vi "中水三立数据传输UI.vi"() -> ()   [LabVIEW 2016, in "中水三立SQL数据传输.lvlib"]
panel:
  in  "开机启动":bool
  out "数据大小":i32
  out "数据上传中":bool
  out "当前时间":timestamp
  out "error out":errorcluster
  out "数据查表起始时间":cluster{"dbo.LS_Data":string}
  in  "数据补传":bool caption="确定"
  out "读取报文显示":string
  out "发送报文显示":string
  out "通信状态":bool
  in  "配置信息":T1
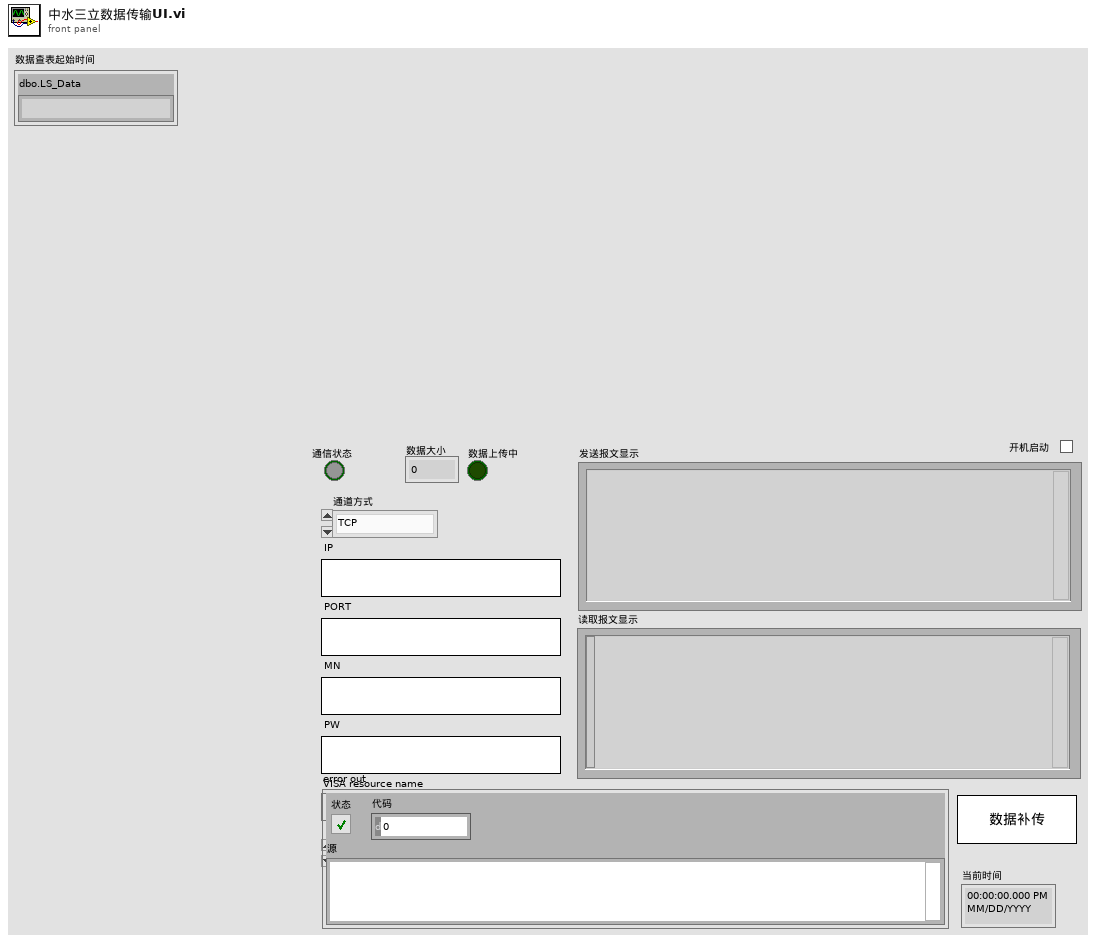
[diagram p1: front panel]
types:
  T1 = cluster{"通道方式":enum16{"TCP", "serial"}, "IP":string, "PORT":string, "MN":string, "PW":string, "VISA resource name":refnum<visa-resource-name>, "baud rate":u32}
  T2 = typedef "LVDateTimeRec.ctl" = cluster{"秒数的小数部分":dbl, "秒":i32, "分":i32, "时":i32, "日":i32, "月":i32, "年":i32, "天数（周）":i32, "天数（年）":i32, "DST":i32}
  T3 = cluster{"枚举":enum16{"打开连接", "发送数据", "读取数据", "数据处理", "关闭连接"}, "data":string}
  T4 = cluster{"枚举":enum16{"TCP", "serial"}, "IP":string, "PORT":string, "MN":string, "PW":string, "VISA resource name":refnum<visa-resource-name>, "baud rate":u32}
  T5 = typedef "中水三立SQL数据传输.lvlib/data_in.ctl" = cluster{"PW":string, "MN":string, "table输入":T6, "数据发送次数":i32, "枚举":enum16{"返回请求应答", "上传数据", "返回执行结果"}, "type":T7, "因子编码&数据类型":cluster{"因子编码":string, "数据类型":string}[]}
  T6 = typedef "中水三立SQL数据传输.lvlib/table.ctl" = string
  T7 = typedef "中水三立SQL数据传输.lvlib/Type.ctl" = string
  T8 = cluster{"table":string, "columns":string[], "condition":string, "data_in":T5}
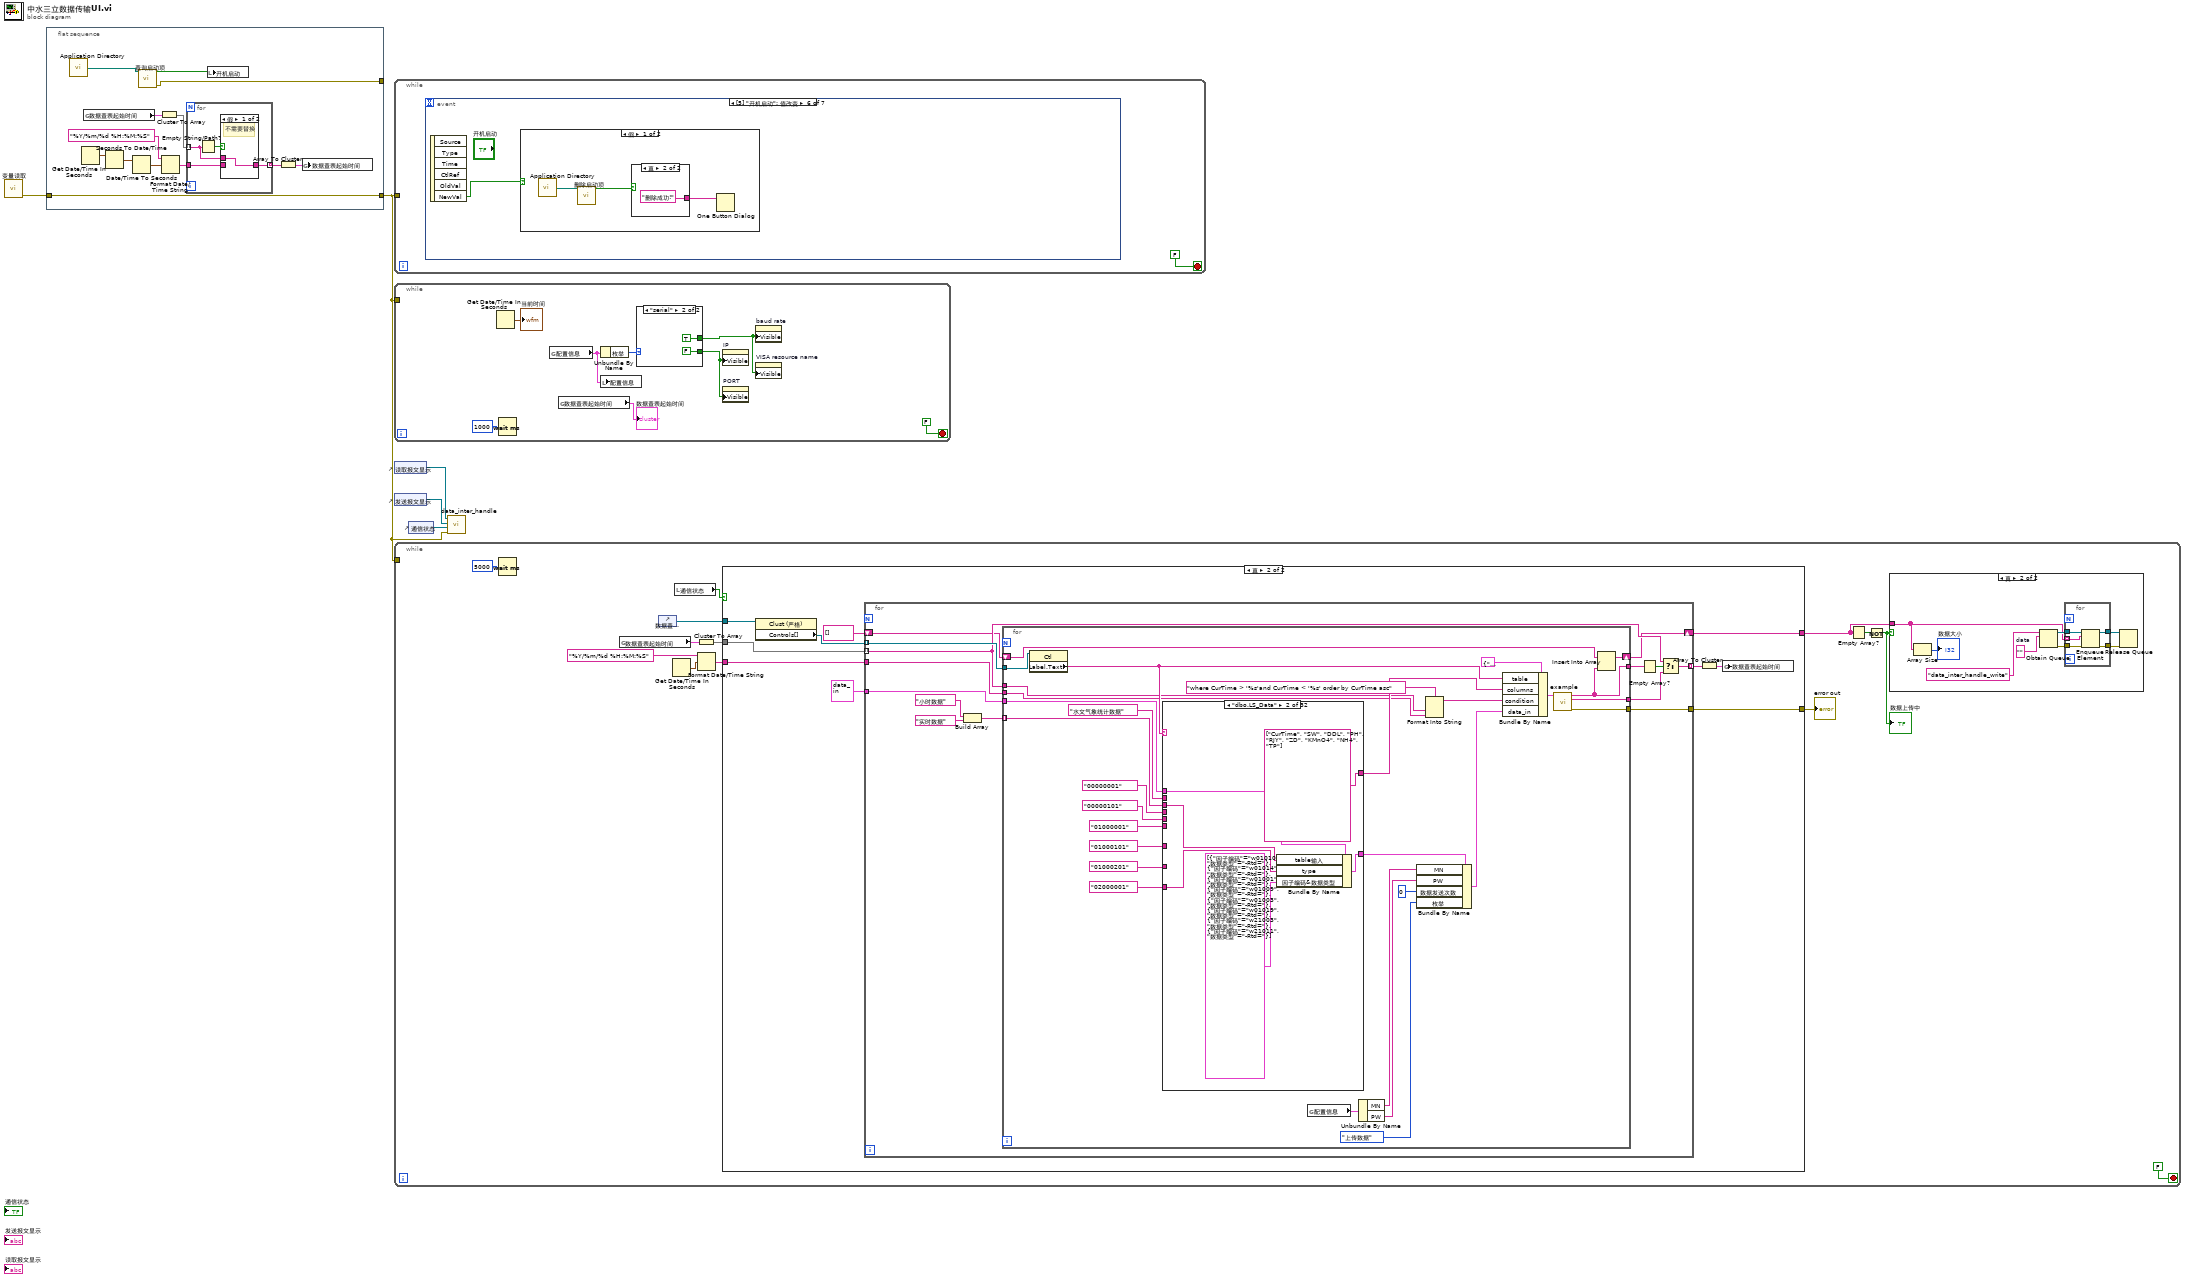
[diagram p0: block diagram]
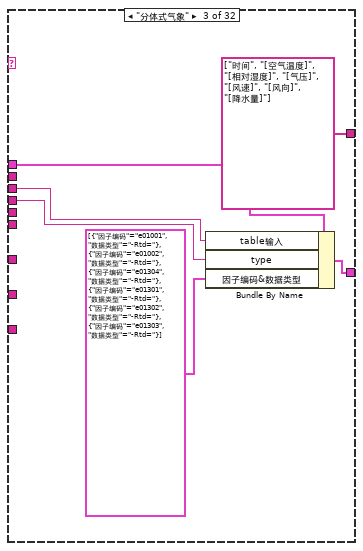
[diagram p5: hidden frame]
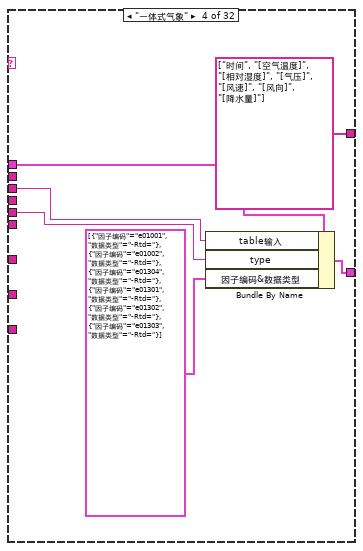
[diagram p6: hidden frame]
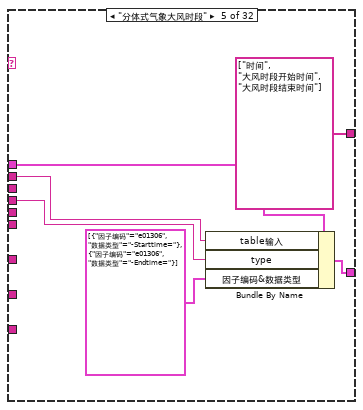
[diagram p7: hidden frame]
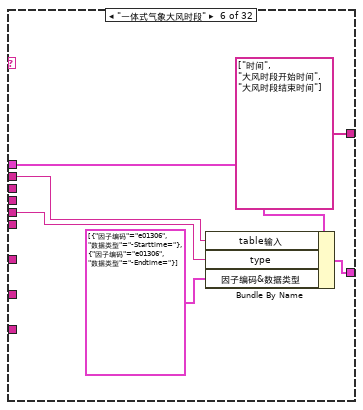
[diagram p8: hidden frame]
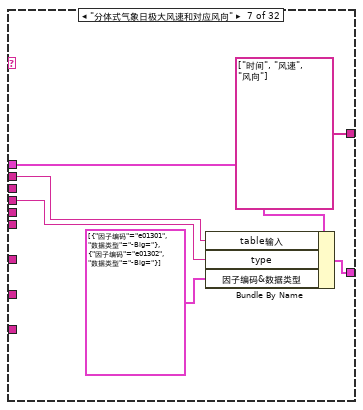
[diagram p9: hidden frame]
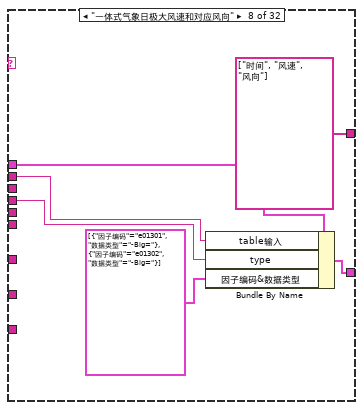
[diagram p10: hidden frame]
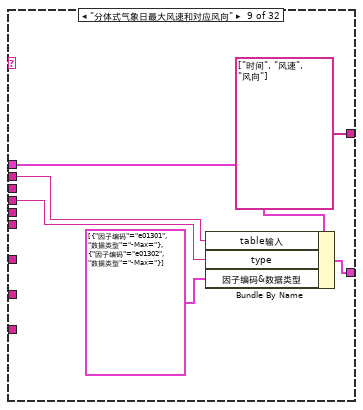
[diagram p11: hidden frame]
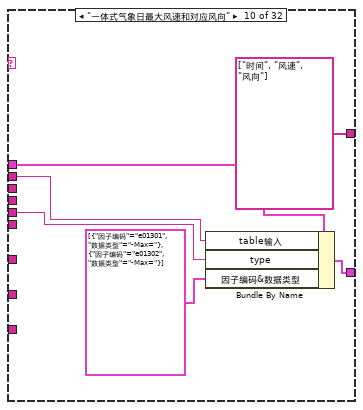
[diagram p12: hidden frame]
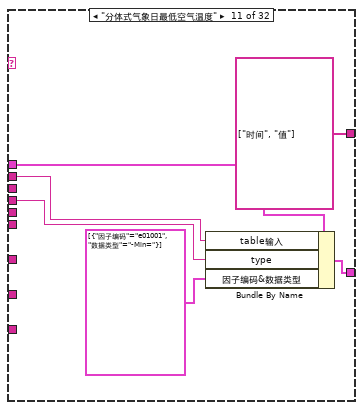
[diagram p13: hidden frame]
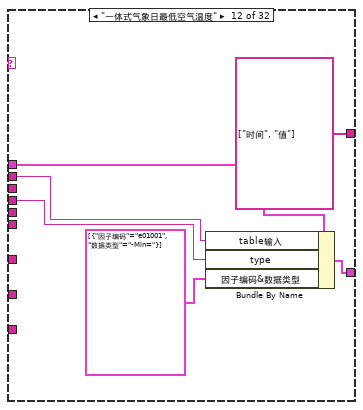
[diagram p14: hidden frame]
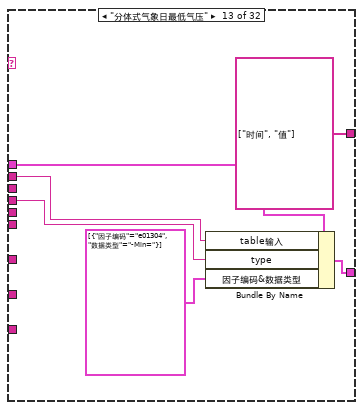
[diagram p15: hidden frame]
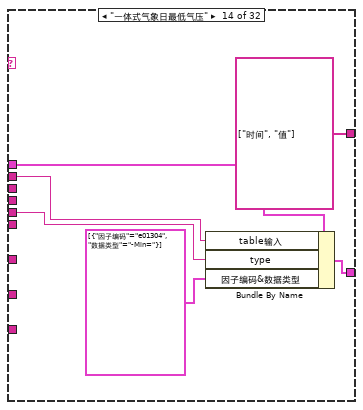
[diagram p16: hidden frame]
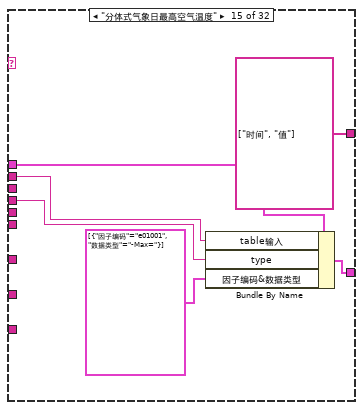
[diagram p17: hidden frame]
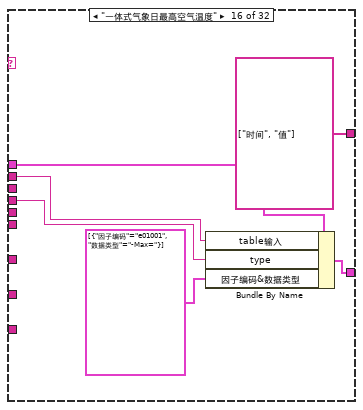
[diagram p18: hidden frame]
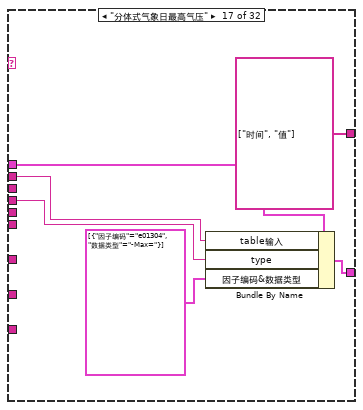
[diagram p19: hidden frame]
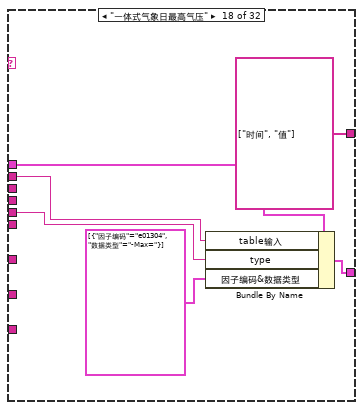
[diagram p20: hidden frame]
diagram:
  n1 = call "变量读取.vi"() -> ("错误输出"=w5:errorcluster)  [unwired: 11 in]
  n2 = flat-sequence {
    tunnel: w5 -> [w11]
    tunnel: [w11] -> w4
    tunnel: [w6] -> _
    frame #0 {
      n3 = call <vilib>:"Application Directory.vi"() -> ("Application Directory"=w8:path)
      n4 = Get Date/Time In Seconds() -> (seconds since 1Jan1904=w10:timestamp)
      n5 = global read "断电保存全局.vi" "数据查表起始时间"() -> (w16:cluster{"dbo.LS_Data":string})
      n6 = Seconds To Date/Time(time stamp (now)=w10) -> (date time rec=w9:T2)  [unwired: 1 in]
      n7 = Date/Time To Seconds(2:w9) -> (0:w14:timestamp)  [unwired: 1 in]
      n8 = call "查询启动项.vi"("启动文件路径"=w8) -> ("error out"=w6:errorcluster, "包含启动项"=w7:bool)  [unwired: 9 in]
      n9 = Cluster To Array(cluster=w16) -> (array=w17:string[])
      n10 = Format Date/Time String(time format string (%c)="%Y/%m/%d %H:%M:%S" ("时间格式字符串(%c)"), seconds (now)=w14) -> (date/time string=w13:string)  [unwired: 1 in]
      n11 = for {
        tunnel: w17 -> [w19] mode=indexing
        tunnel: w13 -> [w21]
        tunnel: [w20] -> w18 mode=indexing
        n12 = Empty String/Path?(string/path=w19) -> (empty?=w22:bool)
        n13 = case shown="假" w22 {
          tunnel: w21 -> [_ w24]
          tunnel: [w23 w24] -> w20
          tunnel: w19 -> [w23 _]
          frame False {
            # "不需要替换"
          }
          frame True {
            # "空字符串，替换"
          }
        }
      }
      n14 = local write "开机启动"(w7) -> ()
      n15 = Array To Cluster(array=w18) -> (cluster=w12:cluster{"[0]":string})
      n16 = global write "断电保存全局.vi" "数据查表起始时间"(w12) -> ()
    }
  }
  n17 = while {
    tunnel: w4 -> [_]
    stop <- FALSE stop-if-true
    n18 = event shown="[5] \"开机启动\": 值改变" {
      selector: _ -> [_ _ _ _ _ _ _]
      dyn-events: _ -> [_ _ _ _ _ _ _]
      timeout: _ -> [_ _ _ _ _ _ _]
      event Timeout {
        n19 = event-data() -> ()  [unwired: 1 in, 3 out]
      }
      event "配置信息.IP", "配置信息.PORT": Mouse Down {
        n20 = event-data() -> ("CtlRef"=w34:refnum<vi>)  [unwired: 1 in, 7 out]
        n21 = property class="Str"(reference=w34) -> (reference out=w27:refnum<vi>, "Value"=w33:string)  [unwired: 1 in, 1 out]
        n22 = call "IP键盘.vi"("OldNumber"=w33) -> ("NewNumber"=w26:string)
        n23 = String Length(string=w26) -> (length=w32:i32)
        n24 = Less Or Equal?(x=w32, y=50) -> (x <= y?=w30:bool)
        n25 = case shown="假" w30 {
          tunnel: w27 -> [w35 w39]
          tunnel: w26 -> [_ w38]
          tunnel: [w35 w39] -> w29
          tunnel: ["127.0.0.1" w38] -> w28
          frame False {
            n26 = One Button Dialog(message="超过ipv4最大长度限制,请重新输入!" ("消息")) -> ()  [unwired: 1 in, 1 out]
          }
          frame True {
          }
        }
        n27 = property class="Str"(reference=w29, "Val(Sgnl)"=w28) -> ()  [unwired: 1 in, 2 out]
      }
      event "配置信息.baud rate": Mouse Down {
        n28 = event-data() -> ("CtlRef"=w43:refnum<vi>)  [unwired: 1 in, 7 out]
        n29 = property class="DigNum (严格)"(reference=w43) -> (reference out=w41:refnum<vi>, "Value"=w42:u32)  [unwired: 1 in, 1 out]
        n30 = call "数字键盘.vi"("OldNumber"=w42) -> ("NewNumber"=w40:sgl)
        n31 = property class="DigNum (严格)"(reference=w41, "Val(Sgnl)"=w40) -> ()  [unwired: 1 in, 2 out]
      }
      event "配置信息": Value Change {
        n32 = event-data() -> ()  [unwired: 1 in, 6 out]
        n33 = flat-sequence {
          frame #0 {
            n34 = global write "断电保存全局.vi" "配置信息"("配置信息") -> ()
          }
          frame #1 {
            w49 = T3 {"枚举"=enum."打开连接", "data"=""}
            n35 = call "变量存储.vi"() -> ()  [unwired: 12 in]
            n36 = Bundle By Name(cluster=w49, "枚举"=enum16{"打开连接", "发送数据", "读取数据", "数据处理", "关闭连接"}."关闭连接") -> (w48:T3)
            n37 = Obtain Queue(name (unnamed)="data_inter_handle" ("名称（未命名）"), element data type=w49) -> (queue out=w51:refnum<queue>, error out=w50:errorcluster)  [unwired: 3 in, 1 out]
            n38 = Enqueue Element(queue=w51, element=w48, error in (no error)=w50) -> (queue out=w45:refnum<queue>, error out=w46:errorcluster)  [unwired: 1 in, 1 out]
            n39 = Release Queue(queue=w45, error in (no error)=w46) -> ()  [unwired: 1 in, 3 out]
          }
        }
      }
      event "数据补传": Value Change {
        n40 = event-data() -> ()  [unwired: 1 in, 6 out]
        n41 = call "数据补传对话框.vi"() -> ("输出"=w54:bool, "时间OUT"=w53:timestamp)  [unwired: 10 in]
        n42 = case shown="真" w54 {
          tunnel: w53 -> [_ w59]
          frame False {
          }
          frame True {
            n43 = Format Date/Time String(time format string (%c)="%Y/%m/%d %H:%M:%S" ("时间格式字符串(%c)"), seconds (now)=w59) -> (date/time string=w56:string)  [unwired: 1 in]
            n44 = Initialize Array(w56, 1 ("维数大小")) -> (w55:string[])
            n45 = Array To Cluster(array=w55) -> (cluster=w57:cluster{"[0]":string})
            n46 = global write "断电保存全局.vi" "数据查表起始时间"(w57) -> ()
          }
        }
      }
      event "开机启动": Value Change {
        n47 = event-data() -> ("NewVal"=w61:bool)  [unwired: 1 in, 5 out]
        n48 = case shown="假" w61 {
          frame False {
            n49 = call <vilib>:"Application Directory.vi"() -> ("Application Directory"=w63:path)
            n50 = call "删除启动项.vi"("启动文件路径"=w63) -> ("删除标记"=w62:bool)  [unwired: 9 in, 1 out]
            n51 = case shown="真" w62 {
              tunnel: ["删除失败!" "删除成功!"] -> w64
              frame False {
              }
              frame True {
              }
            }
            n52 = One Button Dialog(message=w64) -> ()  [unwired: 1 in, 1 out]
          }
          frame True {
            n53 = call <vilib>:"Application Directory.vi"() -> ("Application Directory"=w69:path)
            n54 = call "添加启动项.vi"("启动文件路径"=w69) -> ("添加成功标记"=w68:bool)  [unwired: 9 in, 1 out]
            n55 = case shown="假" w68 {
              tunnel: ["添加失败!" "添加成功!"] -> w67
              frame False {
              }
              frame True {
              }
            }
            n56 = One Button Dialog(message=w67) -> ()  [unwired: 1 in, 1 out]
          }
        }
      }
      event Panel Close {
        n57 = event-data() -> ()  [unwired: 1 in, 4 out]
        n58 = Quit LabVIEW(quit? (T)=TRUE ("退出？(T)")) -> ()
      }
    }
  }
  n59 = while {
    tunnel: w4 -> [_]
    stop <- FALSE stop-if-true
    n60 = Get Date/Time In Seconds() -> (seconds since 1Jan1904=→"当前时间":timestamp)
    n61 = Wait (ms)(milliseconds to wait=u32 1000 ("等待时间（毫秒）")) -> ()  [unwired: 1 out]
    n62 = global read "断电保存全局.vi" "配置信息"() -> (w76:T4)
    n63 = global read "断电保存全局.vi" "数据查表起始时间"() -> (→"数据查表起始时间":cluster{"dbo.LS_Data":string})
    n64 = local write "配置信息"(w76) -> ()
    n65 = Unbundle By Name(w76) -> ("枚举"=w75:enum16{"TCP", "serial"})
    n66 = case shown="\"serial\"" w75 {
      tunnel: [TRUE FALSE] -> w74
      tunnel: [FALSE TRUE] -> w73
      frame "TCP", Default {
      }
      frame "serial" {
      }
    }
    n67 = property on="IP" class="Str"("Visible"=w74) -> ()  [unwired: 2 in, 2 out]
    n68 = property on="PORT" class="Str"("Visible"=w74) -> ()  [unwired: 2 in, 2 out]
    n69 = property on="baud rate" class="DigNum (严格)"("Visible"=w73) -> ()  [unwired: 2 in, 2 out]
    n70 = property on="VISA resource name" class="VISAName"("Visible"=w73) -> ()  [unwired: 2 in, 2 out]
  }
  n71 = control-ref of="读取报文显示"() -> (w2:refnum<vi>)
  n72 = control-ref of="发送报文显示"() -> (w3:refnum<vi>)
  n73 = while {
    tunnel: w4 -> [_]
    stop <- FALSE stop-if-true
    n74 = Wait (ms)(milliseconds to wait=u32 5000 ("等待时间（毫秒）")) -> ()  [unwired: 1 out]
    n75 = global read "断电保存全局.vi" "数据查表起始时间"() -> (w95:cluster{"dbo.LS_Data":string})
    n76 = control-ref of="数据查表起始时间"() -> (w89:refnum<vi>)
    n77 = Get Date/Time In Seconds() -> (seconds since 1Jan1904=w91:timestamp)
    n78 = local read "通信状态"() -> (w86:bool)
    n79 = Cluster To Array(cluster=w95) -> (array=w94:string[])
    n80 = Format Date/Time String(time format string (%c)="%Y/%m/%d %H:%M:%S" ("时间格式字符串(%c)"), seconds (now)=w91) -> (date/time string=w92:string)  [unwired: 1 in]
    n81 = case shown="真" w86 {
      tunnel: w94 -> [_ w107]
      tunnel: w92 -> [_ w106]
      tunnel: [_ w105] -> w85
      tunnel: w89 -> [_ w104]
      tunnel: [_ w102] -> w88
      frame False {
      }
      frame True {
        n82 = property class="Clust (严格)"(reference=w104) -> ("Controls[]"=w103:refnum<vi>[])  [unwired: 1 in, 2 out]
        n83 = for {
          tunnel: w107 -> [w117] mode=indexing
          tunnel: w103 -> [w121] mode=indexing
          tunnel: w106 -> [w120]
          shift-right: [w108] -> w105
          shift-left: string[] [] ("message") -> [w109]
          tunnel: [w115] -> w99 mode=indexing
          tunnel: [w114] -> w102
          tunnel: T5 {"PW"="123456", "MN"="TEST001", "table输入"="心跳包", "数据发送次数"=0, "枚举"=enum."上传数据", "type"="00000001", "因子编码&数据类型"=[{"因子编码"="e01306", "数据类型"="-Starttime="}, {"因子编码"="e01307", "数据类型"="-Endtime="}]} ("data_in") -> [w113]
          n84 = Build Array(T6 "小时数据" ("table输入"), T6 "实时数据" ("table输入")) -> (w110:T6[])
          n85 = for {
            tunnel: w121 -> [w151]
            tunnel: w120 -> [w140]
            tunnel: [w123] -> w119
            tunnel: w117 -> [w138]
            tunnel: [w137] -> w116
            tunnel: [w136] -> w114
            tunnel: w113 -> [w134]
            tunnel: w110 -> [w125] mode=indexing
            shift-right: [w122] -> w108
            shift-left: w109 -> [w124]
            n86 = property class="Ctl"(reference=w151) -> ("Label.Text"=w150:string)  [unwired: 1 in, 2 out]
            n87 = case shown="\"dbo.LS_Data\"" w150 {
              tunnel: [_ string[] ["CurTime", "SW", "DDL", "PH", "RJY", "ZD", "KMnO4", "NH4", "TP"] ("columns") string[] ["时间", "[空气温度]", "[相对湿度]", "[气压]", "[风速]", "[风向]", "[降水量]"] ("columns") string[] ["时间", "[空气温度]", "[相对湿度]", "[气压]", "[风速]", "[风向]", "[降水量]"] ("columns") string[] ["时间", "大风时段开始时间", "大风时段结束时间"] ("columns") string[] ["时间", "大风时段开始时间", "大风时段结束时间"] ("columns") string[] ["时间", "风速", "风向"] ("columns") string[] ["时间", "风速", "风向"] ("columns") string[] ["时间", "风速", "风向"] ("columns") string[] ["时间", "风速", "风向"] ("columns") string[] ["时间", "值"] ("columns") string[] ["时间", "值"] ("columns") string[] ["时间", "值"] ("columns") string[] ["时间", "值"] ("columns") string[] ["时间", "值"] ("columns") string[] ["时间", "值"] ("columns") string[] ["时间", "值"] ("columns") string[] ["时间", "值"] ("columns") string[] ["时间", "值"] ("columns") string[] ["时间", "值"] ("columns") string[] ["时间", "值"] ("columns") string[] ["时间", "值"] ("columns") string[] ["时间", "[60秒能见度]"] ("columns") string[] ["时间", "[潮高]"] ("columns") string[] ["时间", "[潮高]"] ("columns") string[] ["时间", "[潮高]"] ("columns") string[] ["时间", "[潮高]"] ("columns") string[] ["时间", "[潮高]"] ("columns") string[] ["时间", "[潮高]"] ("columns") string[] ["时间", "[潮高]"] ("columns") string[] ["时间", "[潮高]"] ("columns") string[] ["时间", "[潮高]"] ("columns")] -> w149
              tunnel: w134 -> [_ w156 w162 w168 w174 w180 w186 w192 w198 w204 w210 w216 w222 w228 w234 w240 w246 w252 w258 w264 w270 w276 w282 w288 w294 w300 w306 w312 w318 w324 w330 w336]
              tunnel: [_ w155 w161 w167 w173 w179 w185 w191 w197 w203 w209 w215 w221 w227 w233 w239 w245 w251 w257 w263 w269 w275 w281 w287 w293 w299 w305 w311 w317 w323 w329 w335] -> w148
              tunnel: T7 "00000001" ("type") -> [_ _ w158 _ w171 _ w183 w188 w195 _ w207 w213 w219 _ w231 w237 w243 _ w255 _ w266 _ w278 _ _ _ _ _ _ _ _ _]
              tunnel: T7 "00000101" ("type") -> [_ _ _ w164 _ w176 _ _ _ w201 _ _ _ w225 _ _ _ w249 _ w261 _ w273 _ _ _ _ _ _ _ _ _ _]
              tunnel: T7 "01000001" ("type") -> [_ _ _ _ _ _ _ _ _ _ _ _ _ _ _ _ _ _ _ _ _ _ _ w285 _ _ w302 _ _ w321 _ _]
              tunnel: T7 "01000101" ("type") -> [_ _ _ _ _ _ _ _ _ _ _ _ _ _ _ _ _ _ _ _ _ _ _ _ w291 _ _ w309 _ _ w326 _]
              tunnel: T7 "01000201" ("type") -> [_ _ _ _ _ _ _ _ _ _ _ _ _ _ _ _ _ _ _ _ _ _ _ _ _ w297 _ _ w314 _ _ w333]
              tunnel: T7 "02000001" ("type") -> [_ w152 _ _ _ _ _ _ _ _ _ _ _ _ _ _ _ _ _ _ _ _ _ _ _ _ _ _ _ _ _ _]
              tunnel: w125 -> [_ w153 w159 w165 _ _ _ _ _ _ _ _ _ _ _ _ _ _ _ _ _ _ w279 w284 w290 w296 _ _ _ _ _ _]
              tunnel: T6 "水文气象统计数据" ("table输入") -> [_ _ _ _ w170 w177 w182 w189 w194 w200 w206 w212 w218 w224 w230 w236 w242 w248 w254 w260 w267 w272 _ _ _ _ w303 w308 w315 w320 w327 w332]
              frame "假", Default {
              }
              frame "dbo.LS_Data" {
                n88 = Bundle By Name(cluster=w156, "table输入"=w153, "type"=w152, "因子编码&数据类型"=cluster{"因子编码":string, "数据类型":string}[] [{"因子编码"="w01010", "数据类型"="-Rtd="}, {"因子编码"="w01014", "数据类型"="-Rtd="}, {"因子编码"="w01001", "数据类型"="-Rtd="}, {"因子编码"="w01009", "数据类型"="-Rtd="}, {"因子编码"="w01003", "数据类型"="-Rtd="}, {"因子编码"="w01019", "数据类型"="-Rtd="}, {"因子编码"="w21003", "数据类型"="-Rtd="}, {"因子编码"="w21011", "数据类型"="-Rtd="}]) -> (w155:T5)
              }
              frame "分体式气象" {
                n89 = Bundle By Name(cluster=w162, "table输入"=w159, "type"=w158, "因子编码&数据类型"=cluster{"因子编码":string, "数据类型":string}[] [{"因子编码"="e01001", "数据类型"="-Rtd="}, {"因子编码"="e01002", "数据类型"="-Rtd="}, {"因子编码"="e01304", "数据类型"="-Rtd="}, {"因子编码"="e01301", "数据类型"="-Rtd="}, {"因子编码"="e01302", "数据类型"="-Rtd="}, {"因子编码"="e01303", "数据类型"="-Rtd="}]) -> (w161:T5)
              }
              frame "一体式气象" {
                n90 = Bundle By Name(cluster=w168, "table输入"=w165, "type"=w164, "因子编码&数据类型"=cluster{"因子编码":string, "数据类型":string}[] [{"因子编码"="e01001", "数据类型"="-Rtd="}, {"因子编码"="e01002", "数据类型"="-Rtd="}, {"因子编码"="e01304", "数据类型"="-Rtd="}, {"因子编码"="e01301", "数据类型"="-Rtd="}, {"因子编码"="e01302", "数据类型"="-Rtd="}, {"因子编码"="e01303", "数据类型"="-Rtd="}]) -> (w167:T5)
              }
              frame "分体式气象大风时段" {
                n91 = Bundle By Name(cluster=w174, "table输入"=w170, "type"=w171, "因子编码&数据类型"=cluster{"因子编码":string, "数据类型":string}[] [{"因子编码"="e01306", "数据类型"="-Starttime="}, {"因子编码"="e01306", "数据类型"="-Endtime="}]) -> (w173:T5)
              }
              frame "一体式气象大风时段" {
                n92 = Bundle By Name(cluster=w180, "table输入"=w177, "type"=w176, "因子编码&数据类型"=cluster{"因子编码":string, "数据类型":string}[] [{"因子编码"="e01306", "数据类型"="-Starttime="}, {"因子编码"="e01306", "数据类型"="-Endtime="}]) -> (w179:T5)
              }
              frame "分体式气象日极大风速和对应风向" {
                n93 = Bundle By Name(cluster=w186, "table输入"=w182, "type"=w183, "因子编码&数据类型"=cluster{"因子编码":string, "数据类型":string}[] [{"因子编码"="e01301", "数据类型"="-Big="}, {"因子编码"="e01302", "数据类型"="-Big="}]) -> (w185:T5)
              }
              frame "一体式气象日极大风速和对应风向" {
                n94 = Bundle By Name(cluster=w192, "table输入"=w189, "type"=w188, "因子编码&数据类型"=cluster{"因子编码":string, "数据类型":string}[] [{"因子编码"="e01301", "数据类型"="-Big="}, {"因子编码"="e01302", "数据类型"="-Big="}]) -> (w191:T5)
              }
              frame "分体式气象日最大风速和对应风向" {
                n95 = Bundle By Name(cluster=w198, "table输入"=w194, "type"=w195, "因子编码&数据类型"=cluster{"因子编码":string, "数据类型":string}[] [{"因子编码"="e01301", "数据类型"="-Max="}, {"因子编码"="e01302", "数据类型"="-Max="}]) -> (w197:T5)
              }
              frame "一体式气象日最大风速和对应风向" {
                n96 = Bundle By Name(cluster=w204, "table输入"=w200, "type"=w201, "因子编码&数据类型"=cluster{"因子编码":string, "数据类型":string}[] [{"因子编码"="e01301", "数据类型"="-Max="}, {"因子编码"="e01302", "数据类型"="-Max="}]) -> (w203:T5)
              }
              frame "分体式气象日最低空气温度" {
                n97 = Bundle By Name(cluster=w210, "table输入"=w206, "type"=w207, "因子编码&数据类型"=cluster{"因子编码":string, "数据类型":string}[] [{"因子编码"="e01001", "数据类型"="-Min="}]) -> (w209:T5)
              }
              frame "一体式气象日最低空气温度" {
                n98 = Bundle By Name(cluster=w216, "table输入"=w212, "type"=w213, "因子编码&数据类型"=cluster{"因子编码":string, "数据类型":string}[] [{"因子编码"="e01001", "数据类型"="-Min="}]) -> (w215:T5)
              }
              frame "分体式气象日最低气压" {
                n99 = Bundle By Name(cluster=w222, "table输入"=w218, "type"=w219, "因子编码&数据类型"=cluster{"因子编码":string, "数据类型":string}[] [{"因子编码"="e01304", "数据类型"="-Min="}]) -> (w221:T5)
              }
              frame "一体式气象日最低气压" {
                n100 = Bundle By Name(cluster=w228, "table输入"=w224, "type"=w225, "因子编码&数据类型"=cluster{"因子编码":string, "数据类型":string}[] [{"因子编码"="e01304", "数据类型"="-Min="}]) -> (w227:T5)
              }
              frame "分体式气象日最高空气温度" {
                n101 = Bundle By Name(cluster=w234, "table输入"=w230, "type"=w231, "因子编码&数据类型"=cluster{"因子编码":string, "数据类型":string}[] [{"因子编码"="e01001", "数据类型"="-Max="}]) -> (w233:T5)
              }
              frame "一体式气象日最高空气温度" {
                n102 = Bundle By Name(cluster=w240, "table输入"=w236, "type"=w237, "因子编码&数据类型"=cluster{"因子编码":string, "数据类型":string}[] [{"因子编码"="e01001", "数据类型"="-Max="}]) -> (w239:T5)
              }
              frame "分体式气象日最高气压" {
                n103 = Bundle By Name(cluster=w246, "table输入"=w242, "type"=w243, "因子编码&数据类型"=cluster{"因子编码":string, "数据类型":string}[] [{"因子编码"="e01304", "数据类型"="-Max="}]) -> (w245:T5)
              }
              frame "一体式气象日最高气压" {
                n104 = Bundle By Name(cluster=w252, "table输入"=w248, "type"=w249, "因子编码&数据类型"=cluster{"因子编码":string, "数据类型":string}[] [{"因子编码"="e01304", "数据类型"="-Max="}]) -> (w251:T5)
              }
              frame "分体式气象日最小相对湿度" {
                n105 = Bundle By Name(cluster=w258, "table输入"=w254, "type"=w255, "因子编码&数据类型"=cluster{"因子编码":string, "数据类型":string}[] [{"因子编码"="e01002", "数据类型"="-Min="}]) -> (w257:T5)
              }
              frame "一体式气象日最小相对湿度" {
                n106 = Bundle By Name(cluster=w264, "table输入"=w260, "type"=w261, "因子编码&数据类型"=cluster{"因子编码":string, "数据类型":string}[] [{"因子编码"="e01002", "数据类型"="-Min="}]) -> (w263:T5)
              }
              frame "分体式气象日降水量" {
                n107 = Bundle By Name(cluster=w270, "table输入"=w267, "type"=w266, "因子编码&数据类型"=cluster{"因子编码":string, "数据类型":string}[] [{"因子编码"="e01303", "数据类型"="-Day="}]) -> (w269:T5)
              }
              frame "一体式气象日降水量" {
                n108 = Bundle By Name(cluster=w276, "table输入"=w272, "type"=w273, "因子编码&数据类型"=cluster{"因子编码":string, "数据类型":string}[] [{"因子编码"="e01303", "数据类型"="-Day="}]) -> (w275:T5)
              }
              frame "能见度" {
                n109 = Bundle By Name(cluster=w282, "table输入"=w279, "type"=w278, "因子编码&数据类型"=cluster{"因子编码":string, "数据类型":string}[] [{"因子编码"="e01305", "数据类型"="-Rtd="}]) -> (w281:T5)
              }
              frame "浮子水位计" {
                n110 = Bundle By Name(cluster=w288, "table输入"=w284, "type"=w285, "因子编码&数据类型"=cluster{"因子编码":string, "数据类型":string}[] [{"因子编码"="e01308", "数据类型"="-Rtd="}]) -> (w287:T5)
              }
              frame "雷达水位计" {
                n111 = Bundle By Name(cluster=w294, "table输入"=w290, "type"=w291, "因子编码&数据类型"=cluster{"因子编码":string, "数据类型":string}[] [{"因子编码"="e01308", "数据类型"="-Rtd="}]) -> (w293:T5)
              }
              frame "压力水位计" {
                n112 = Bundle By Name(cluster=w300, "table输入"=w296, "type"=w297, "因子编码&数据类型"=cluster{"因子编码":string, "数据类型":string}[] [{"因子编码"="e01308", "数据类型"="-Rtd="}]) -> (w299:T5)
              }
              frame "浮子水位计低潮" {
                n113 = Bundle By Name(cluster=w306, "table输入"=w303, "type"=w302, "因子编码&数据类型"=cluster{"因子编码":string, "数据类型":string}[] [{"因子编码"="e01310", "数据类型"="-Trough="}]) -> (w305:T5)
              }
              frame "雷达水位计低潮" {
                n114 = Bundle By Name(cluster=w312, "table输入"=w308, "type"=w309, "因子编码&数据类型"=cluster{"因子编码":string, "数据类型":string}[] [{"因子编码"="e01310", "数据类型"="-Trough="}]) -> (w311:T5)
              }
              frame "压力水位计低潮" {
                n115 = Bundle By Name(cluster=w318, "table输入"=w315, "type"=w314, "因子编码&数据类型"=cluster{"因子编码":string, "数据类型":string}[] [{"因子编码"="e01310", "数据类型"="-Trough="}]) -> (w317:T5)
              }
              frame "浮子水位计高潮" {
                n116 = Bundle By Name(cluster=w324, "table输入"=w320, "type"=w321, "因子编码&数据类型"=cluster{"因子编码":string, "数据类型":string}[] [{"因子编码"="e01309", "数据类型"="-Peak="}]) -> (w323:T5)
              }
              frame "雷达水位计高潮" {
                n117 = Bundle By Name(cluster=w330, "table输入"=w327, "type"=w326, "因子编码&数据类型"=cluster{"因子编码":string, "数据类型":string}[] [{"因子编码"="e01309", "数据类型"="-Peak="}]) -> (w329:T5)
              }
              frame "压力水位计高潮" {
                n118 = Bundle By Name(cluster=w336, "table输入"=w332, "type"=w333, "因子编码&数据类型"=cluster{"因子编码":string, "数据类型":string}[] [{"因子编码"="e01309", "数据类型"="-Peak="}]) -> (w335:T5)
              }
            }
            n119 = global read "断电保存全局.vi" "配置信息"() -> (w147:T4)
            n120 = Unbundle By Name(w147) -> ("MN"=w146:string, "PW"=w145:string)
            n121 = Bundle By Name(cluster=w148, "MN"=w146, "PW"=w145, "数据发送次数"=0, "枚举"=enum16{"返回请求应答", "上传数据", "返回执行结果"}."上传数据") -> (w142:T5)
            n122 = Format Into String(format string="where CurTime > '%s'and CurTime < '%s' order by CurTime asc" ("初始字符串"), w138, w140) -> (resulting string=w139:string)  [unwired: 2 in, 1 out]
            n123 = Bundle By Name(cluster=T8 {"table"="分体式气象大风时段", "columns"=["时间", "大风时段开始时间", "大风时段结束时间"], "condition"="", "data_in"={"PW"="123456", "MN"="TEST001", "table输入"="心跳包", "数据发送次数"=0, "枚举"=enum."上传数据", "type"="00000001", "因子编码&数据类型"=[{"因子编码"="e01306", "数据类型"="-Starttime="}, {"因子编码"="e01307", "数据类型"="-Endtime="}]}} ("data_in"), "table"=w150, "columns"=w149, "condition"=w139, "data_in"=w142) -> (w126:T8)
            n124 = call "example.vi"("data_in"=w126) -> ("error out"=w136:errorcluster, "最新时间"=w137:string, "message"=w123:string[])  [unwired: 8 in]
            n125 = Insert Into Array(array=w124, new element=w123) -> (w122:string[])  [unwired: 1 in]
          }
          n126 = Empty Array?(array=w119) -> (empty?=w118:bool)
          n127 = Select(t=w117, s=w118, f=w116) -> (s? t:f=w115:string)
        }
        n128 = Array To Cluster(array=w99) -> (cluster=w100:cluster{"[0]":string})
        n129 = global write "断电保存全局.vi" "数据查表起始时间"(w100) -> ()
      }
    }
    "error out" <- w88
    n130 = Empty Array?(array=w85) -> (empty?=w90:bool)
    n131 = Not(x=w90) -> (.not. x?=w87:bool)
    "数据上传中" <- w87
    n132 = case shown="真" w87 {
      tunnel: w85 -> [_ w338]
      frame False {
      }
      frame True {
        w340 = ""  # data
        n133 = Array Size(array=w338) -> (size(s)=→"数据大小":i32)
        n134 = Obtain Queue(name (unnamed)="data_inter_handle_write" ("名称（未命名）"), element data type=w340) -> (queue out=w345:refnum<queue>, error out=w344:errorcluster)  [unwired: 3 in, 1 out]
        n135 = for {
          tunnel: w345 -> [w350]
          tunnel: w344 -> [w349]
          tunnel: [w348] -> w343
          tunnel: [w347] -> w342
          tunnel: w338 -> [w346] mode=indexing
          n136 = Enqueue Element(queue=w350, element=w346, error in (no error)=w349) -> (queue out=w348:refnum<queue>, error out=w347:errorcluster)  [unwired: 1 in, 1 out]
        }
        n137 = Release Queue(queue=w343, error in (no error)=w342) -> ()  [unwired: 1 in, 3 out]
      }
    }
  }
  n138 = control-ref of="通信状态"() -> (w1:refnum<vi>)
  n139 = call "data_inter_handle.vi"("error in (no error)"=w4, "通信状态"=w1, "发送报文显示"=w3, "读取报文显示"=w2) -> ()  [unwired: 7 in, 1 out]
